vi "py File Name.vi"(0 "Path":path, 11 "error in (no error)":errorcluster) -> (4 "Doc Name":string, 6 "Shell Name":string, 15 "error out":errorcluster)   [LabVIEW 2016, in "Py Doc.lvclass"]
uses:
  Py Doc.lvclass
  <vilib>/regexp/Match Regular Expression.xnode
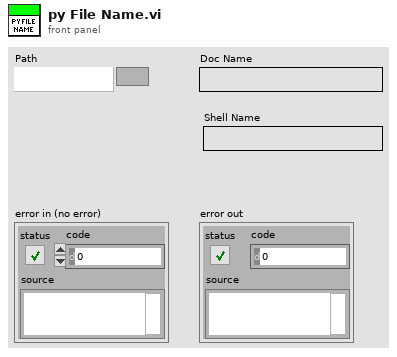
[diagram p1: front panel]
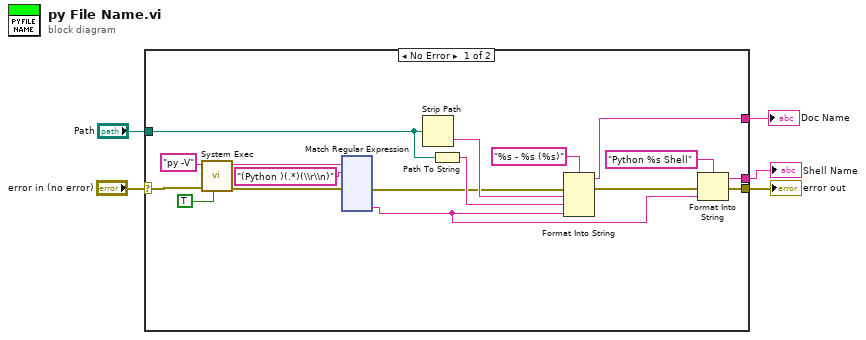
[diagram p0: block diagram]
diagram:
  n1 = case shown="No Error" "error in (no error)" {
    selector: "error in (no error)" -> [w16 w140]
    tunnel: "Path" -> [w22 _]
    tunnel: [w20 _] -> w4
    tunnel: [w14 w140] -> w2
    tunnel: [w11 _] -> w1
    frame No Error {
      n2 = call <vilib>:"System Exec.vi"("run minimized? (F)"=TRUE, "error in (no error)"=w16, "command line"="py -V") -> ("error out"=w7:errorcluster, "standard output"=w8:string)  [unwired: 5 in, 2 out]
      n3 = xnode "Match Regular Expression"("input string"=w8, "regular expression"="(Python )(.*)(\\r\\n)", "error in"=w7) -> ("error out"=w15:errorcluster, "submatch 2"=w12:string)  [unwired: 3 in, 5 out]
      n4 = Strip Path(path=w22) -> (name=w18:string)  [unwired: 1 out]
      n5 = Path To String(path=w22) -> (string=w21:string)
      n6 = Format Into String(format string="%s - %s (%s)", error in=w15, w18, w21, w12) -> (resulting string=w20:string, error out=w17:errorcluster)  [unwired: 1 in]
      n7 = Format Into String(format string="Python %s Shell", error in=w17, w12) -> (resulting string=w11:string, error out=w14:errorcluster)  [unwired: 1 in]
    }
    frame Error {
    }
  }
  "Doc Name" <- w4
  "error out" <- w2
  "Shell Name" <- w1
